vi "custom error read.vi"() -> (0 "Description":string[](array[string]), 1 "Codes":i32[](array[numeric]), 2 "file or folder exists?":bool)   [LabVIEW 2010, in "ErrorLog.lvlib"]
doc: "This VI reads the error information (codes and descriptions) from a file that can be used to add custom error information to ADCPro.\n\nInputs:\nPath - path of the file if not using the default error file (default is custom_errors.txt located in the same place as this VI.\nAuto - boolean to use default file and location or user specified file and location\n\nOutputs:"
uses:
  ErrorLog.lvlib
panel:
  in  "Default":bool=TRUE
  in  "Path":path
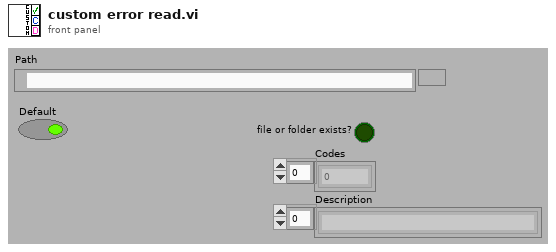
[diagram p1: front panel]
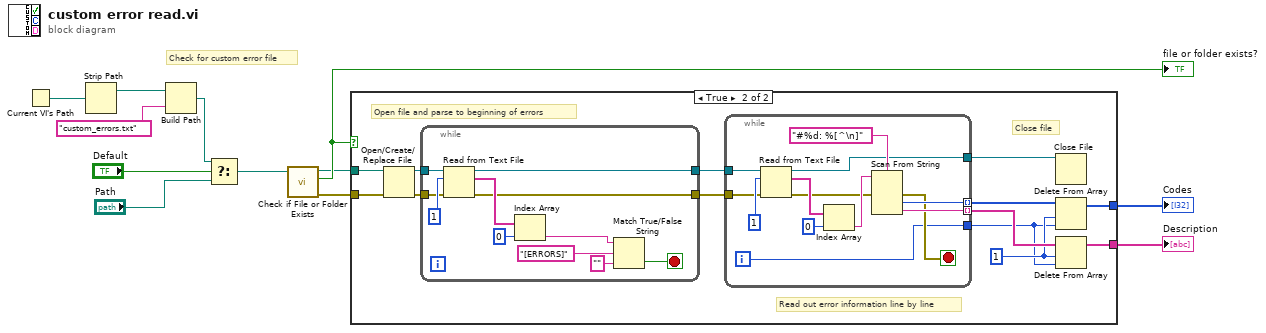
[diagram p0: block diagram]
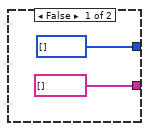
[diagram p2: hidden frame]
diagram:
  # "Check for custom error file"
  n1 = Current VI's Path() -> (path=w5:path)
  n2 = Strip Path(path=w5) -> (stripped path=w4:path)  [unwired: 1 out]
  n3 = Build Path(base path=w4, name or relative path="custom_errors.txt") -> (appended path=w2:path)
  n4 = Select(t=w2, s="Default", f="Path") -> (s? t:f=w6:path)
  n5 = call <vilib>:"Check if File or Folder Exists.vi"("path"=w6) -> ("error out"=w10:errorcluster, "file or folder exists?"=w12:bool, "dup path"=w11:path)  [unwired: 8 in]
  "file or folder exists?" <- w12
  n6 = case shown="True" w12 {
    tunnel: w11 -> [_ w27]
    tunnel: w10 -> [_ w26]
    tunnel: [i32[] [] w16] -> w8
    tunnel: [string[] [] w15] -> w9
    frame False {
    }
    frame True {
      w18 = 1
      # "Close file"
      # "Read out error information line by line"
      # "Open file and parse to beginning of errors"
      n7 = Open/Create/Replace File(file path (use dialog)=w27, error in=w26) -> (refnum out=w24:refnum<file>, error out=w25:errorcluster)  [unwired: 4 in, 1 out]
      n8 = while {
        tunnel: w25 -> [w50]
        tunnel: w24 -> [w49]
        tunnel: [w41] -> w23
        tunnel: [w42] -> w22
        stop <- w44 stop-if-true
        n9 = Read from Text File(file (use dialog)=w49, count=1, error in=w50) -> (refnum out=w42:refnum<file>, text=w47:string[], error out=w41:errorcluster)  [unwired: 1 in, 1 out]
        n10 = Index Array(array=w47, index=0) -> (element=w45:string)
        n11 = Match True/False String(2:"" ("false string"), 3:"[ERRORS]" ("string"), 4:w45) -> (0:w44:bool)  [unwired: 1 out]
      }
      n12 = while {
        tunnel: w23 -> [w28]
        tunnel: w22 -> [w29]
        tunnel: [w38] -> w21
        tunnel: [w33] -> w20 mode=indexing
        tunnel: [w32] -> w19 mode=indexing
        tunnel: [w30] -> w17
        i -> [w30]
        stop <- w31 stop-if-true
        n13 = Read from Text File(file (use dialog)=w29, count=1, error in=w28) -> (refnum out=w38:refnum<file>, text=w35:string[], error out=w34:errorcluster)  [unwired: 1 in, 1 out]
        n14 = Index Array(array=w35, index=0) -> (element=w36:string)
        n15 = Scan From String(format string="#%d: %[^\n]", input string=w36, error in=w34) -> (error out=w31:errorcluster, output 1=w33:i32, output 2=w32:string)  [unwired: 3 in, 2 out]
      }
      n16 = Close File(refnum=w21) -> ()  [unwired: 1 in, 2 out]
      n17 = Delete From Array(array=w20, length=w18, index=w17) -> (array with subset deleted=w16:i32[])  [unwired: 1 out]
      n18 = Delete From Array(array=w19, length=w18, index=w17) -> (array with subset deleted=w15:string[])  [unwired: 1 out]
    }
  }
  "Codes" <- w8
  "Description" <- w9
